vi "DB Open.vi"(8 "error in":errorcluster, 10 "DB":T1={"DataSource Name"="eDCU_LTT", "userID"="root", "password"="edultt"}, 11 "Database in":refnum<class "SQLite Database.lvclass">) -> (0 "error out":errorcluster, 3 "Database out":refnum<class "SQLite Database.lvclass">)   [LabVIEW 2023, in "HardwareAbstractionLayer_LVOOP.lvlib" / "SQLite Database.lvclass"]
doc: "This VI is Database Connection Open"
uses:
  SQLite Database.lvclass
  SQLite Database.lvclass/SQLite Database.ctl
  <vilib>/addons/database/Connection.llb/DB Tools Open Connec (String).vi
  <vilib>/addons/database/NI_Database_API.lvlib
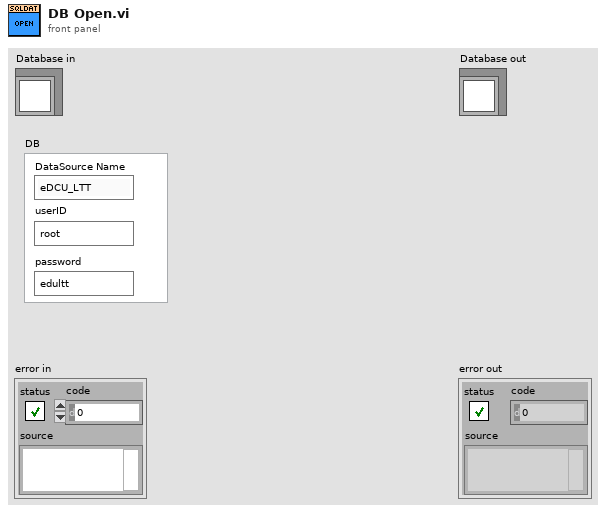
[diagram p1: front panel]
types:
  T1 = cluster{"DataSource Name":string, "userID":string, "password":string}
  T2 = typedef "NI_Database_API.lvlib/Conn ObjectReference.ctl" = refnum<k1>
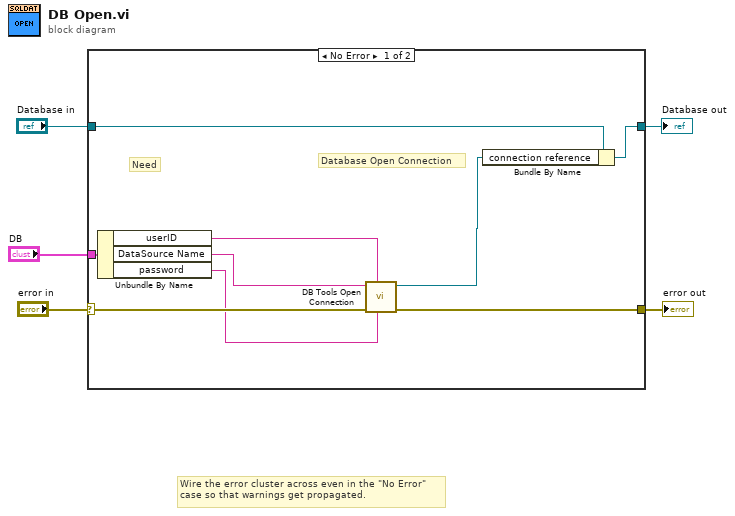
[diagram p0: block diagram]
diagram:
  # "Wire the error cluster across even in the \"No Error\"\ncase so that warnings get propagated."
  n1 = case shown="No Error" "error in" {
    selector: "error in" -> [w14 w16]
    tunnel: [w13 w16] -> w4
    tunnel: [w8 w15] -> w2
    tunnel: "Database in" -> [w9 w15]
    tunnel: "DB" -> [w6 _]
    frame No Error {
      # "Need"
      # "Database Open Connection"
      n2 = Unbundle By Name(w6) -> ("userID"=w12:string, "DataSource Name"=w11:string, "password"=w10:string)
      n3 = call-poly <vilib>:"DB Tools Open Connection.vi"("password"=w10, "userID"=w12, "error in (no error)"=w14, "connection information"=w11) -> ("error out"=w13:errorcluster, "connection reference"=w7:T2)  [unwired: 4 in]
      n4 = Bundle By Name(cluster=w9, "connection reference"=w7) -> (w8:refnum<class "SQLite Database.lvclass">)
    }
    frame Error {
    }
  }
  "error out" <- w4
  "Database out" <- w2
